vi "dropNode.vi"(8 "error in (no error)":errorcluster, 9 "Drop Node Path":string, 10 "Drag Node Path":string, 11 "xceRootNode in":refnum<class "xceRootNode.lvclass">) -> (0 "error out":errorcluster, 3 "xceRootNode out":refnum<class "xceRootNode.lvclass">)   [LabVIEW 2013, in "xceRootNode.lvclass"]
doc: "Used in a drag/drop operation, when the user has detrmined where in the tree control they would like to drop."
uses:
  xceRootNode.lvclass
  xceDataNode/xceDataNode.lvclass
  xceRootNode.lvclass/xceRootNode.ctl
  xceNode/xceNode.lvclass
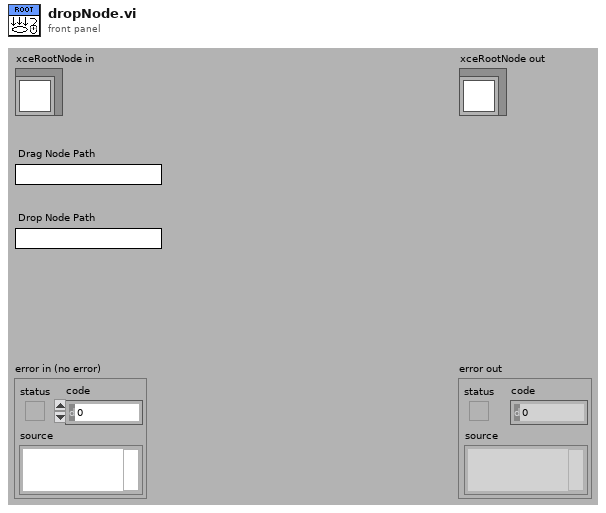
[diagram p1: front panel]
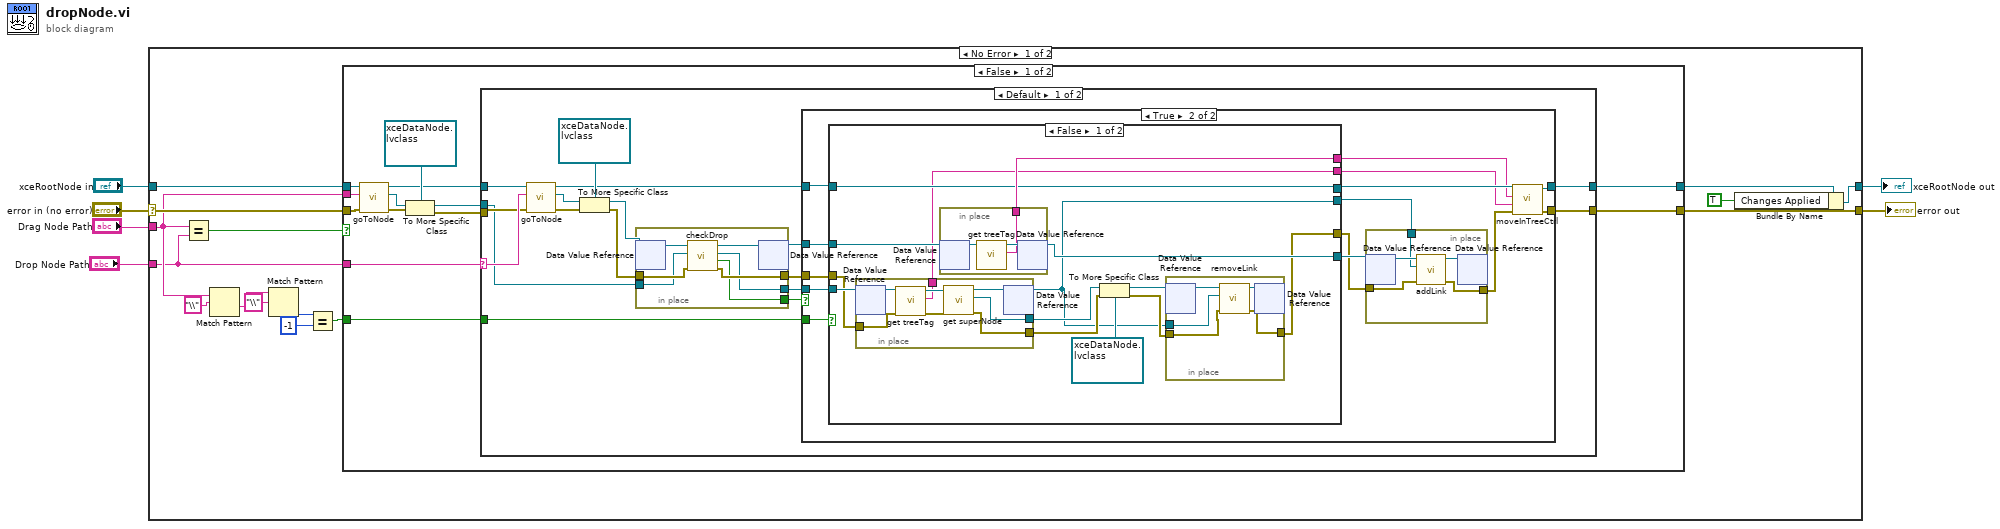
[diagram p0: block diagram]
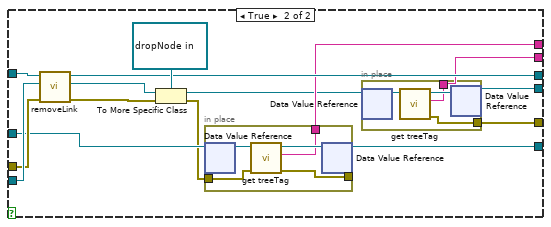
[diagram p3: hidden frame]
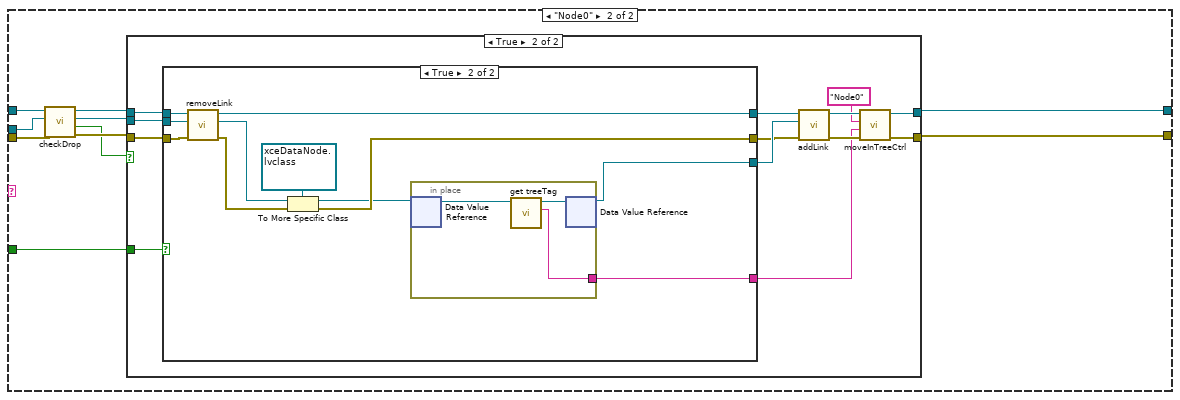
[diagram p4: hidden frame]
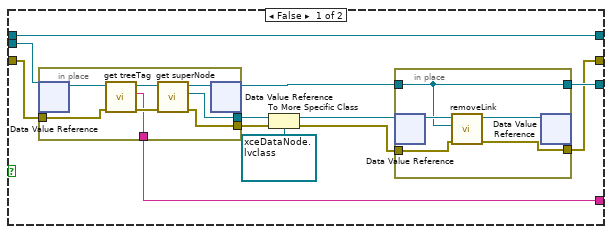
[diagram p6: hidden frame]
diagram:
  n1 = case shown="No Error" "error in (no error)" {
    selector: "error in (no error)" -> [w20 w200]
    tunnel: [w18 w200] -> w5
    tunnel: [w8 w199] -> w3
    tunnel: "xceRootNode in" -> [w21 w199]
    tunnel: "Drag Node Path" -> [w12 _]
    tunnel: "Drop Node Path" -> [w11 _]
    frame No Error {
      n2 = Equal?(x=w12, y=w11) -> (x = y?=w19:bool)
      n3 = Match Pattern(string=w12, regular expression="\\") -> (after substring=w14:string)  [unwired: 1 in, 3 out]
      n4 = Match Pattern(string=w14, regular expression="\\") -> (offset past match=w16:i32)  [unwired: 1 in, 3 out]
      n5 = Equal?(x=w16, y=-1) -> (x = y?=w10:bool)
      n6 = case shown="False" w19 {
        tunnel: w21 -> [w34 w198]
        tunnel: w20 -> [w33 w197]
        tunnel: w12 -> [w28 _]
        tunnel: w11 -> [w27 _]
        tunnel: [w26 w198] -> w9
        tunnel: [w25 w197] -> w18
        tunnel: w10 -> [w22 _]
        frame False {
          n7 = call "goToNode.vi"("error in (no error)"=w33, "Node Path"=w28, "xceNode in"=w34) -> ("error out"=w31:errorcluster, "goToNode* out"=w32:refnum<data-value>, "xceNode out"=w29:refnum<class "xceRootNode.lvclass">)  [unwired: 6 in]
          n8 = To More Specific Class(target class=refnum<data-value> refnum ("data value reference"), reference=w32, error in=w31) -> (specific class reference=w23:refnum<data-value>, error out=w24:errorcluster)
          n9 = case shown="Default" w27 {
            selector: w27 -> [w50 _]
            tunnel: w29 -> [w51 w142]
            tunnel: [w40 w137] -> w26
            tunnel: [w38 w134] -> w25
            tunnel: w24 -> [w49 w141]
            tunnel: w23 -> [w43 w139]
            tunnel: w22 -> [w36 w135]
            frame Default {
              n10 = call "goToNode.vi"("error in (no error)"=w49, "Node Path"=w50, "xceNode in"=w51) -> ("error out"=w46:errorcluster, "goToNode* out"=w47:refnum<data-value>, "xceNode out"=w41:refnum<class "xceRootNode.lvclass">)  [unwired: 6 in]
              n11 = To More Specific Class(target class=refnum<data-value> refnum ("data value reference"), reference=w47, error in=w46) -> (specific class reference=w45:refnum<data-value>, error out=w44:errorcluster)
              n12 = in-place {
                in-place-border: w44 -> [w131]
                in-place-border: w43 -> [w130]
                in-place-border: [w129] -> w39
                in-place-border: [w128] -> w37
                in-place-border: [w127] -> w42
                n13 = in-place-dvr #1(w45) -> (w133:refnum<class "xceDataNode.lvclass">)  [unwired: 1 out]
                n14 = call "checkDrop.vi"("error in (no error)"=w131, "dragNode in"=w130, "dropNode in"=w133) -> ("error out"=w129:errorcluster, "validDrop"=w127:bool, "dragNode out"=w128:refnum<data-value>, "dropNode out"=w132:refnum<class "xceDataNode.lvclass">)  [unwired: 5 in]
                n15 = in-place-dvr #1(w132) -> (w35:refnum<data-value>)  [unwired: 1 out]
              }
              n16 = case shown="True" w42 {
                tunnel: w41 -> [w53 w65]
                tunnel: [w53 w61] -> w40
                tunnel: w39 -> [w52 w64]
                tunnel: [w52 w60] -> w38
                tunnel: w37 -> [_ w66]
                tunnel: w36 -> [_ w67]
                tunnel: w35 -> [_ w63]
                frame False {
                }
                frame True {
                  n17 = case shown="False" w67 {
                    tunnel: w66 -> [w86 w116]
                    tunnel: w65 -> [w76 w117]
                    tunnel: w64 -> [w85 w115]
                    tunnel: w63 -> [w80 w112]
                    tunnel: [w76 w109] -> w62
                    tunnel: [w77 w108] -> w57
                    tunnel: [w79 w107] -> w55
                    tunnel: [w73 w106] -> w54
                    tunnel: [w78 w104] -> w59
                    tunnel: [w74 w103] -> w58
                    frame False {
                      n18 = in-place {
                        in-place-border: w85 -> [w97]
                        in-place-border: [w101] -> w84
                        in-place-border: [w100] -> w83
                        in-place-border: [w96] -> w73
                        n19 = in-place-dvr #2(w86) -> (w99:refnum<class "xceDataNode.lvclass">)  [unwired: 1 out]
                        n20 = call "get treeTag.vi"("error in (no error)"=w97, "xceNode in"=w99) -> ("error out"=w95:errorcluster, "treeTag"=w96:string, "xceNode out"=w98:refnum<class "xceDataNode.lvclass">)  [unwired: 7 in]
                        n21 = call "get superNode.vi"("error in (no error)"=w95, "xceNode in"=w98) -> ("error out"=w100:errorcluster, "superNode*"=w101:refnum<data-value>, "xceNode out"=w102:refnum<class "xceDataNode.lvclass">)  [unwired: 7 in]
                        n22 = in-place-dvr #2(w102) -> (w74:refnum<data-value>)  [unwired: 1 out]
                      }
                      n23 = in-place {
                        in-place-border: [w87] -> w79
                        n24 = in-place-dvr #3(w80) -> (w89:refnum<class "xceDataNode.lvclass">)  [unwired: 1 out]
                        n25 = call "get treeTag.vi"("xceNode in"=w89) -> ("treeTag"=w87:string, "xceNode out"=w88:refnum<class "xceDataNode.lvclass">)  [unwired: 8 in, 1 out]
                        n26 = in-place-dvr #3(w88) -> (w78:refnum<data-value>)  [unwired: 1 out]
                      }
                      n27 = To More Specific Class(target class=refnum<data-value> refnum ("data value reference"), reference=w84, error in=w83) -> (specific class reference=w75:refnum<data-value>, error out=w81:errorcluster)
                      n28 = in-place {
                        in-place-border: w74 -> [w92]
                        in-place-border: w81 -> [w91]
                        in-place-border: [w90] -> w77
                        n29 = in-place-dvr #4(w75) -> (w94:refnum<class "xceDataNode.lvclass">)  [unwired: 1 out]
                        n30 = call "removeLink.vi"("error in (no error)"=w91, "subNode in"=w92, "superNode in"=w94) -> ("error out"=w90:errorcluster, "superNode out"=w93:refnum<class "xceDataNode.lvclass">)  [unwired: 6 in, 1 out]
                        n31 = in-place-dvr #4(w93) -> ()  [unwired: 2 out]
                      }
                    }
                    frame True {
                      n32 = call "removeLink.vi"("error in (no error)"=w115, "subNode in"=w116, "superNode in"=w117) -> ("error out"=w113:errorcluster, "subNode out"=w114:refnum<data-value>, "superNode out"=w109:refnum<class "xceRootNode.lvclass">)  [unwired: 6 in]
                      n33 = To More Specific Class(target class=refnum<data-value> refnum ("dragNode out"), reference=w114, error in=w113) -> (specific class reference=w105:refnum<data-value>, error out=w111:errorcluster)
                      n34 = in-place {
                        in-place-border: w111 -> [w122]
                        in-place-border: [w125] -> _
                        in-place-border: [w124] -> w107
                        n35 = in-place-dvr #5(w112) -> (w123:refnum<class "xceDataNode.lvclass">)  [unwired: 1 out]
                        n36 = call "get treeTag.vi"("error in (no error)"=w122, "xceNode in"=w123) -> ("error out"=w125:errorcluster, "treeTag"=w124:string, "xceNode out"=w126:refnum<class "xceDataNode.lvclass">)  [unwired: 7 in]
                        n37 = in-place-dvr #5(w126) -> (w104:refnum<data-value>)  [unwired: 1 out]
                      }
                      n38 = in-place {
                        in-place-border: [w119] -> w108
                        in-place-border: [w118] -> w106
                        n39 = in-place-dvr #6(w105) -> (w121:refnum<class "xceDataNode.lvclass">)  [unwired: 1 out]
                        n40 = call "get treeTag.vi"("xceNode in"=w121) -> ("error out"=w119:errorcluster, "treeTag"=w118:string, "xceNode out"=w120:refnum<class "xceDataNode.lvclass">)  [unwired: 8 in]
                        n41 = in-place-dvr #6(w120) -> (w103:refnum<data-value>)  [unwired: 1 out]
                      }
                    }
                  }
                  n42 = in-place {
                    in-place-border: w58 -> [w71]
                    in-place-border: w57 -> [w70]
                    in-place-border: [w69] -> w56
                    n43 = in-place-dvr #7(w59) -> (w72:refnum<class "xceDataNode.lvclass">)  [unwired: 1 out]
                    n44 = call "addLink.vi"("error in (no error)"=w70, "subNode in"=w71, "superNode in"=w72) -> ("error out"=w69:errorcluster, "superNode out"=w68:refnum<class "xceDataNode.lvclass">)  [unwired: 6 in, 1 out]
                    n45 = in-place-dvr #7(w68) -> ()  [unwired: 2 out]
                  }
                  n46 = call "moveInTreeCtrl.vi"("error in (no error)"=w56, "subNode tag"=w54, "superNode tag"=w55, "xceRootNode in"=w62) -> ("error out"=w60:errorcluster, "xceRootNode out"=w61:refnum<class "xceRootNode.lvclass">)  [unwired: 6 in]
                }
              }
            }
            frame "Node0" {
              n47 = call "checkDrop.vi"("error in (no error)"=w141, "dragNode in"=w139, "dropNode in"=w142) -> ("error out"=w140:errorcluster, "validDrop"=w136:bool, "dropNode out"=w138:refnum<class "xceRootNode.lvclass">)  [unwired: 5 in, 1 out]
              n48 = case shown="True" w136 {
                tunnel: w138 -> [w144 w157]
                tunnel: w140 -> [w143 w156]
                tunnel: w139 -> [_ w155]
                tunnel: [w144 w149] -> w137
                tunnel: w135 -> [_ w154]
                tunnel: [w143 w147] -> w134
                frame False {
                }
                frame True {
                  n49 = case shown="True" w154 {
                    tunnel: w157 -> [w167 w193]
                    tunnel: w156 -> [w168 w192]
                    tunnel: w155 -> [w169 w191]
                    tunnel: [w167 w190] -> w153
                    tunnel: [w160 w184] -> w152
                    tunnel: [w159 w186] -> w151
                    tunnel: [w158 w183] -> w146
                    frame False {
                      n50 = in-place {
                        in-place-border: w168 -> [w176]
                        in-place-border: [w181] -> w166
                        in-place-border: [w180] -> w165
                        in-place-border: [w175] -> w158
                        n51 = in-place-dvr #8(w169) -> (w177:refnum<class "xceDataNode.lvclass">)  [unwired: 1 out]
                        n52 = call "get treeTag.vi"("error in (no error)"=w176, "xceNode in"=w177) -> ("error out"=w178:errorcluster, "treeTag"=w175:string, "xceNode out"=w179:refnum<class "xceDataNode.lvclass">)  [unwired: 7 in]
                        n53 = call "get superNode.vi"("error in (no error)"=w178, "xceNode in"=w179) -> ("error out"=w180:errorcluster, "superNode*"=w181:refnum<data-value>, "xceNode out"=w182:refnum<class "xceDataNode.lvclass">)  [unwired: 7 in]
                        n54 = in-place-dvr #8(w182) -> (w161:refnum<data-value>)  [unwired: 1 out]
                      }
                      n55 = To More Specific Class(target class=refnum<data-value> refnum ("data value reference"), reference=w166, error in=w165) -> (specific class reference=w163:refnum<data-value>, error out=w162:errorcluster)
                      n56 = in-place {
                        in-place-border: w162 -> [w173]
                        in-place-border: w161 -> [w170]
                        in-place-border: [w171] -> w159
                        in-place-border: [w170] -> w160
                        n57 = in-place-dvr #9(w163) -> (w174:refnum<class "xceDataNode.lvclass">)  [unwired: 1 out]
                        n58 = call "removeLink.vi"("error in (no error)"=w173, "subNode in"=w170, "superNode in"=w174) -> ("error out"=w171:errorcluster, "superNode out"=w172:refnum<class "xceDataNode.lvclass">)  [unwired: 6 in, 1 out]
                        n59 = in-place-dvr #9(w172) -> ()  [unwired: 2 out]
                      }
                    }
                    frame True {
                      n60 = call "removeLink.vi"("error in (no error)"=w192, "subNode in"=w191, "superNode in"=w193) -> ("error out"=w187:errorcluster, "subNode out"=w189:refnum<data-value>, "superNode out"=w190:refnum<class "xceRootNode.lvclass">)  [unwired: 6 in]
                      n61 = To More Specific Class(target class=refnum<data-value> refnum ("data value reference"), reference=w189, error in=w187) -> (specific class reference=w185:refnum<data-value>, error out=w186:errorcluster)
                      n62 = in-place {
                        in-place-border: [w194] -> w183
                        n63 = in-place-dvr #10(w185) -> (w196:refnum<class "xceDataNode.lvclass">)  [unwired: 1 out]
                        n64 = call "get treeTag.vi"("xceNode in"=w196) -> ("treeTag"=w194:string, "xceNode out"=w195:refnum<class "xceDataNode.lvclass">)  [unwired: 8 in, 1 out]
                        n65 = in-place-dvr #10(w195) -> (w184:refnum<data-value>)  [unwired: 1 out]
                      }
                    }
                  }
                  n66 = call "addLink.vi"("error in (no error)"=w151, "subNode in"=w152, "superNode in"=w153) -> ("error out"=w148:errorcluster, "superNode out"=w150:refnum<class "xceRootNode.lvclass">)  [unwired: 6 in, 1 out]
                  n67 = call "moveInTreeCtrl.vi"("error in (no error)"=w148, "subNode tag"=w146, "superNode tag"="Node0", "xceRootNode in"=w150) -> ("error out"=w147:errorcluster, "xceRootNode out"=w149:refnum<class "xceRootNode.lvclass">)  [unwired: 6 in]
                }
              }
            }
          }
        }
        frame True {
        }
      }
      n68 = Bundle By Name(cluster=w9, "Changes Applied"=TRUE) -> (w8:refnum<class "xceRootNode.lvclass">)
    }
    frame Error {
    }
  }
  "error out" <- w5
  "xceRootNode out" <- w3
